vi "ConfigInputIncubate.vi"(1 "MulticolumnListbox in":refnum<vi>, 3 "ItemNames in":string[][](array[string])) -> (0 "ItemNames out":string[][](array[string]))   [LabVIEW 2018, in "Config.lvlib"]
uses:
  Config.lvlib
  ContinuousLoop/ContinousLoop.lvlib
panel:
  in  "Replace":bool
  in  "Insert":bool
  in  "Append":bool
  in  "Time":dbl=1.0 min=1.0 step=1.0 format="%<%H:%M:%S>t"
  # "Incubate"
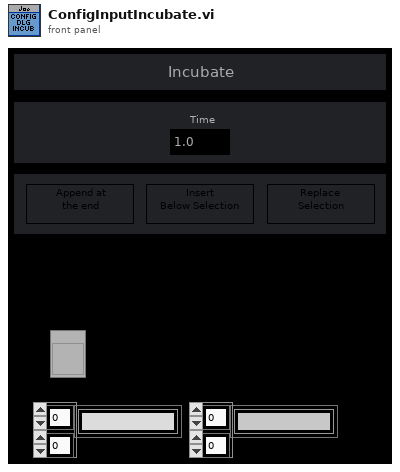
[diagram p1: front panel]
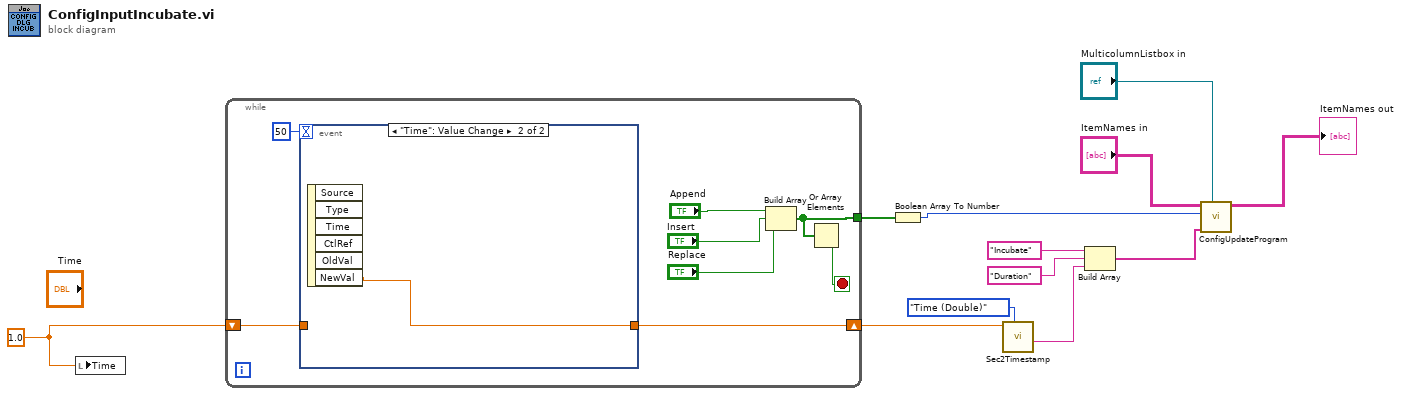
[diagram p0: block diagram]
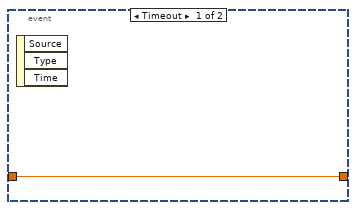
[diagram p2: hidden frame]
diagram:
  w1 = 1.0 ("Mixing Cycles")
  n1 = local write "Time"(w1) -> ()
  n2 = while {
    tunnel: [w15] -> w12
    shift-right: [w14] -> w4
    shift-left: w1 -> [w13]
    stop <- w16 stop-if-true
    n3 = event shown="[1] \"Time\": Value Change" {
      selector: _ -> [_ _]
      dyn-events: _ -> [_ _]
      timeout: 50 -> [_ _]
      tunnel: [w21 w22] -> w14
      tunnel: w13 -> [w21 _]
      event Timeout {
        n4 = event-data() -> ()  [unwired: 1 in, 3 out]
      }
      event "Time": Value Change {
        n5 = event-data() -> ("NewVal"=w22:dbl)  [unwired: 1 in, 5 out]
      }
    }
    n6 = Build Array("Append", "Insert", "Replace") -> (w15:bool[])
    n7 = Or Array Elements(Boolean array=w15) -> (logical OR=w16:bool)
  }
  n8 = Boolean Array To Number(Boolean array=w12) -> (number=w11:u32)
  n9 = call "Sec2Timestamp.vi"("Input Selection"=enum32{"Time (Double)", "Time (Time Stamp)"}."Time (Double)", "Input Time (Double)"=w4) -> ("date/time string"=w3:string)  [unwired: 7 in, 2 out]
  n10 = Build Array("Incubate", "Duration", w3) -> (w2:string[])
  n11 = call "ConfigUpdateProgram.vi"("MulticolumnListbox in"="MulticolumnListbox in", "New Element"=w2, "Operation"=w11, "ItemNames in"="ItemNames in") -> ("ItemNames out"=→"ItemNames out":string[][])  [unwired: 7 in]
